vi "Receiver UI.vi"(8 "Error In":errorcluster) -> (0 "Error Out":errorcluster, 11 "Notification":bool)   [LabVIEW 2020, in "Receiver.lvclass"]
doc: "The VI receives data from sender and displays the received message of different data types."
uses:
  Receiver.lvclass
  Controls/Queue Operation.ctl
  Controls/User Event Operations.ctl
  Controls/Receiver Data.ctl
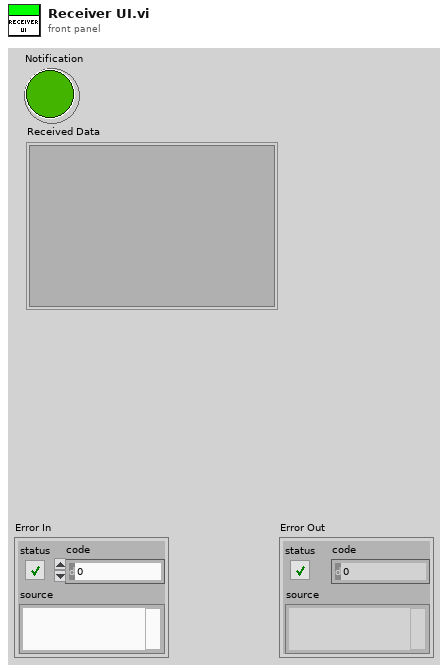
[diagram p1: front panel]
types:
  T1 = typedef "Receiver Data.ctl" = cluster{"Notification":bool}
  T2 = typedef "User Event Operations.ctl" = enum16{"Obtain", "Generate", "Destroy"}
  T3 = typedef "Queue Operation.ctl" = enum16{"Create & Enqueue N", "Enqueue N", "Dequeue", "Enstack N", "Flush", "Release"}
  T4 = typedef "Queue Element.ctl" = cluster{"State":string, "Data":variant}
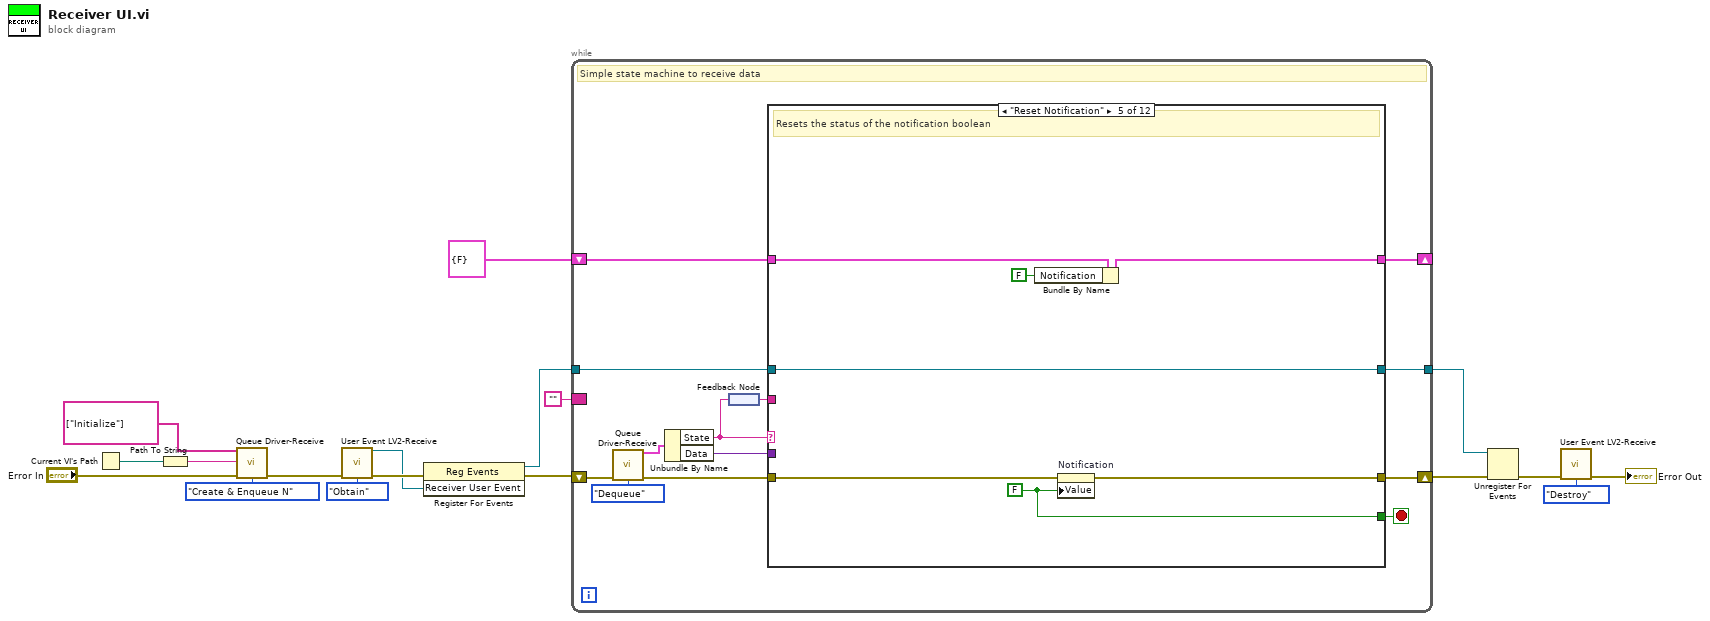
[diagram p0: block diagram]
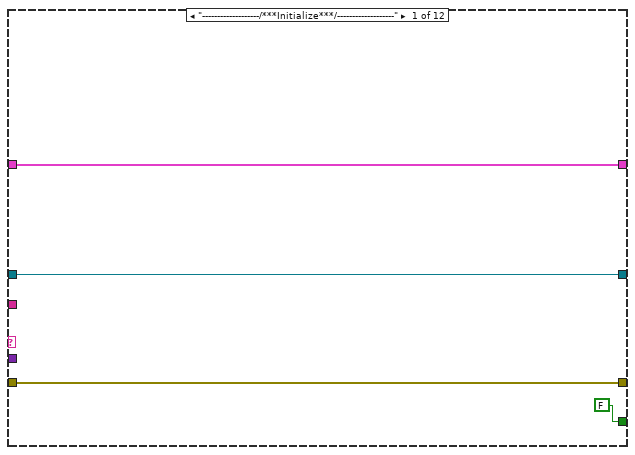
[diagram p2: hidden frame]
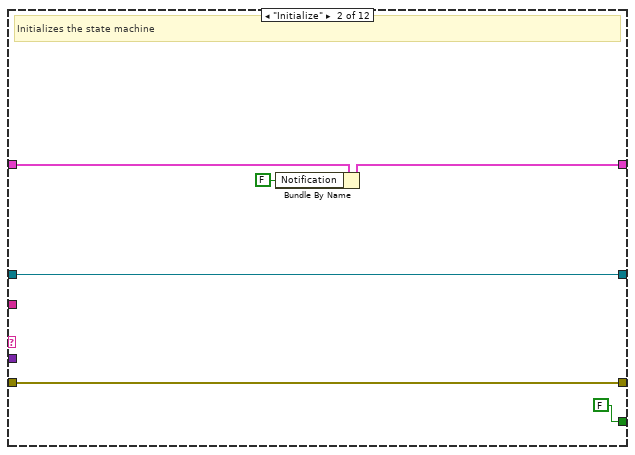
[diagram p3: hidden frame]
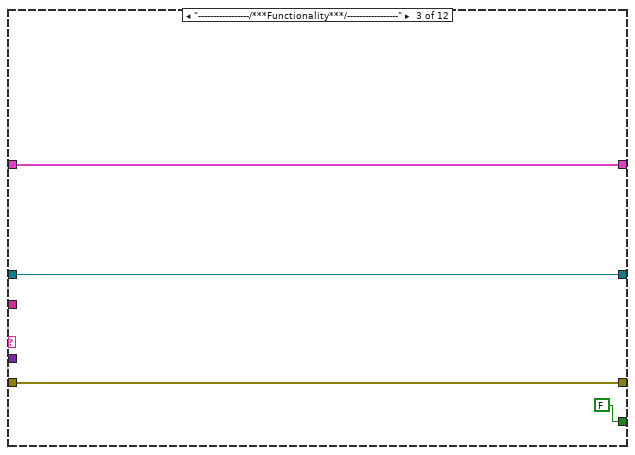
[diagram p4: hidden frame]
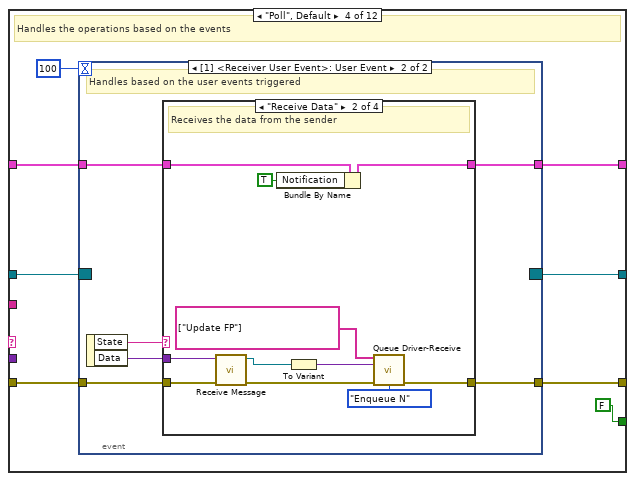
[diagram p5: hidden frame]
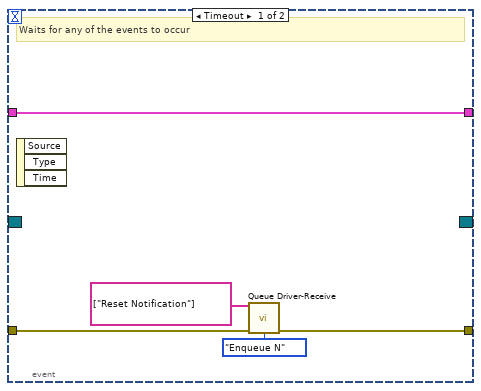
[diagram p6: hidden frame]
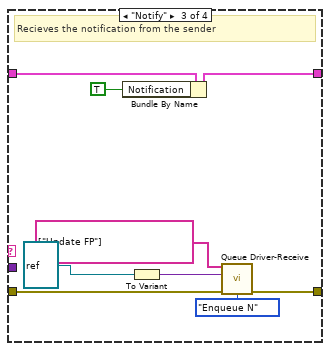
[diagram p8: hidden frame]
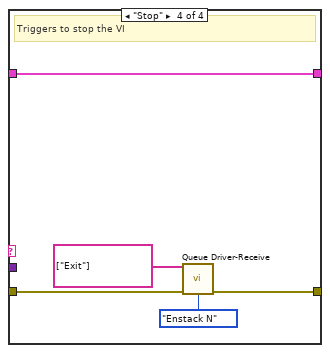
[diagram p9: hidden frame]
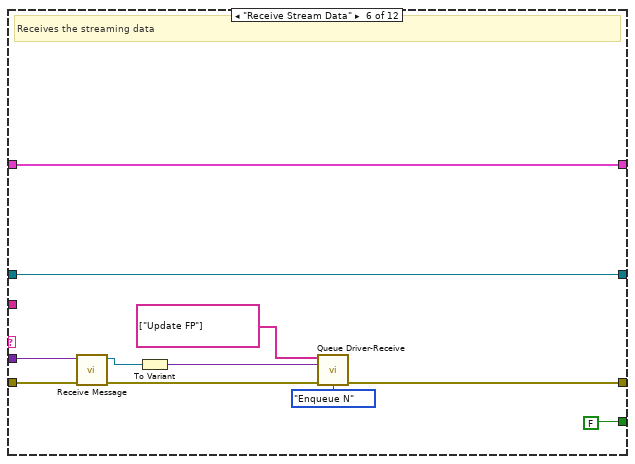
[diagram p10: hidden frame]
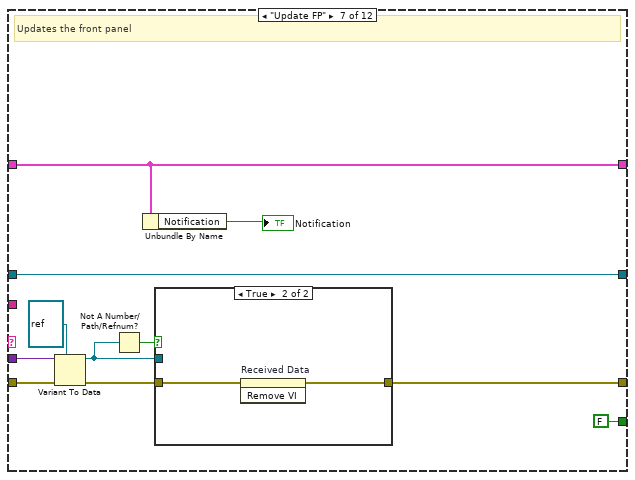
[diagram p11: hidden frame]
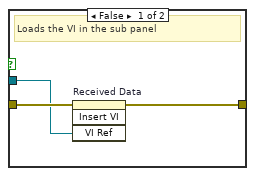
[diagram p12: hidden frame]
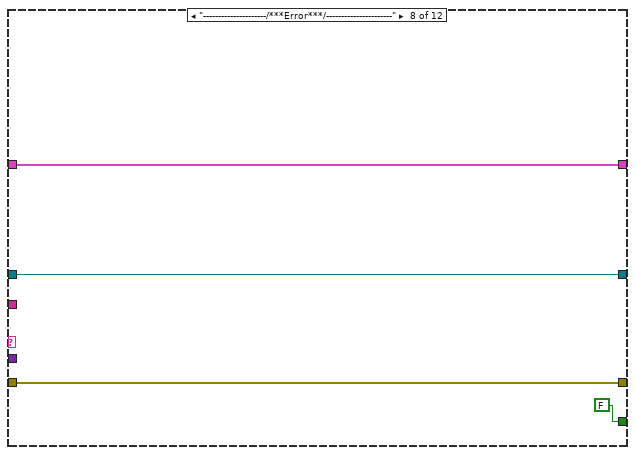
[diagram p13: hidden frame]
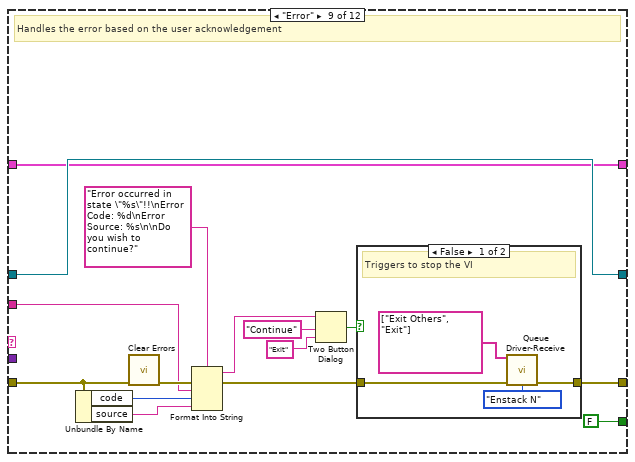
[diagram p14: hidden frame]
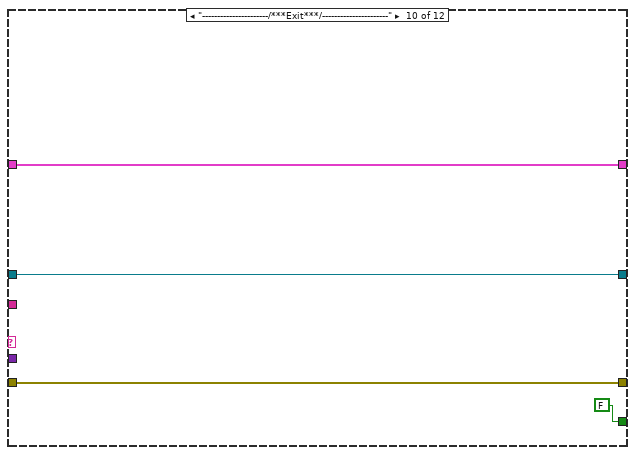
[diagram p16: hidden frame]
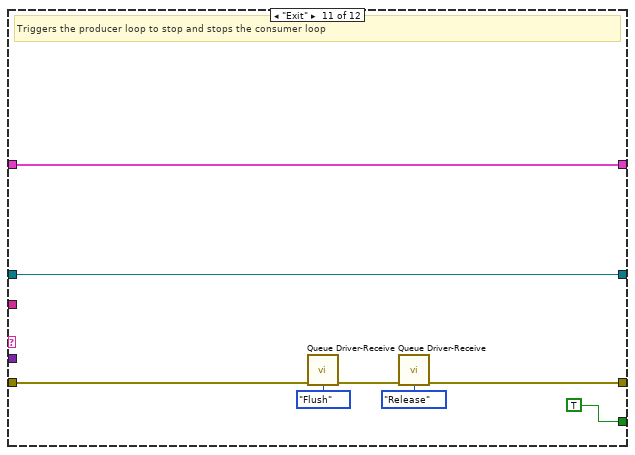
[diagram p17: hidden frame]
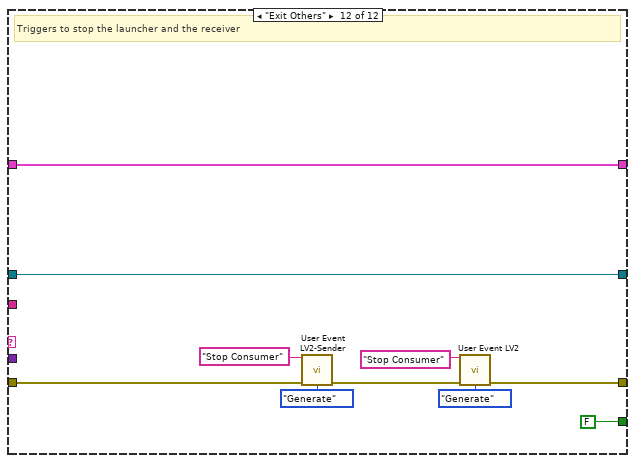
[diagram p18: hidden frame]
diagram:
  n1 = Current VI's Path() -> (path=w3:path)
  n2 = Path To String(path=w3) -> (string=w2:string)
  n3 = call "Queue Driver-Receive.vi"("States[]"=string[] ["Initialize"], "Queue Name"=w2, "Error In"="Error In", "Queue Operation"=Queue_Operation."Create & Enqueue N") -> ("Error Out"=w15:errorcluster)  [unwired: 10 in, 1 out]
  n4 = call "User Event LV2-Receive.vi"("Error In"=w15, "Operation"=User_Event_Operations."Obtain") -> ("Receiver User Event"=w9:refnum<user-event>, "Error Out"=w12:errorcluster)  [unwired: 12 in]
  n5 = register-events(error in=w12, w9) -> (reference out=w8:refnum<event-registration>, error out=w10:errorcluster)  [unwired: 1 in]
  n6 = while {
    shift-right: [w30] -> w16
    shift-left: w10 -> [w31]
    border: "" -> [_]
    tunnel: w8 -> [w23]
    tunnel: [w22] -> w6
    shift-right: [w19] -> _
    shift-left: T1 {"Notification"=FALSE} ("Receiver Data") -> [w20]
    stop <- w27 stop-if-true
    # "Simple state machine to receive data"
    n7 = call "Queue Driver-Receive.vi"("Error In"=w31, "Queue Operation"=Queue_Operation."Dequeue") -> ("Dequeue Element"=w21:T4, "Error Out"=w29:errorcluster)  [unwired: 12 in]
    n8 = Unbundle By Name(w21) -> ("State"=w26:string, "Data"=w24:variant)
    n9 = feedback-in #1(w26) -> ()
    n10 = feedback #1() -> (w25:string)
    n11 = case shown="\"Reset Notification\"" w26 {
      tunnel: w29 -> [w35 w40 w45 w53 w98 w104 w118 w129 w136 w153 w161 w171]
      tunnel: [w35 w40 w45 w51 w96 w107 w117 w129 w133 w153 w157 w166] -> w30
      tunnel: [FALSE FALSE FALSE FALSE w95 FALSE FALSE FALSE FALSE FALSE TRUE FALSE ("Notification")] -> w27
      tunnel: w25 -> [_ _ _ _ _ _ _ _ w134 _ _ _]
      tunnel: w24 -> [_ _ _ _ _ w102 w115 _ _ _ _ _]
      tunnel: w23 -> [w33 w39 w43 w49 w97 w108 w119 w127 w131 w151 w155 w170]
      tunnel: [w33 w39 w43 w48 w97 w108 w119 w127 w131 w151 w155 w170] -> w22
      tunnel: w20 -> [w32 w38 w42 w47 w94 w99 w111 w126 w130 w150 w154 w162]
      tunnel: [w32 w37 w42 w46 w93 w99 w111 w126 w130 w150 w154 w162] -> w19
      frame "-------------------/***Initialize***/-------------------" {
      }
      frame "Initialize" {
        # "Initializes the state machine"
        n12 = Bundle By Name(cluster=w38, "Notification"=FALSE) -> (w37:T1)
      }
      frame "-----------------/***Functionality***/-----------------" {
      }
      frame "Poll", Default {
        # "Handles the operations based on the events"
        n13 = event shown="[1] <Receiver User Event>: User Event" {
          selector: w49 -> [_ _]
          dyn-events: [_ _] -> w48
          timeout: 100 -> [_ _]
          tunnel: w53 -> [w58 w64]
          tunnel: [w57 w63] -> w51
          tunnel: w47 -> [w54 w60]
          tunnel: [w54 w59] -> w46
          event Timeout {
            # "Waits for any of the events to occur"
            n14 = event-data() -> ()  [unwired: 1 in, 3 out]
            n15 = call "Queue Driver-Receive.vi"("States[]"=string[] ["Reset Notification"], "Error In"=w58, "Queue Operation"=Queue_Operation."Enqueue N") -> ("Error Out"=w57:errorcluster)  [unwired: 11 in, 1 out]
          }
          event User Event {
            # "Handles based on the user events triggered"
            n16 = event-data() -> ("State"=w62:string, "Data"=w61:variant)  [unwired: 1 in]
            n17 = case shown="\"Receive Data\"" w62 {
              tunnel: w64 -> [w66 w77 w86 w91]
              tunnel: [w66 w74 w85 w90] -> w63
              tunnel: w61 -> [_ w75 _ _]
              tunnel: w60 -> [w65 w69 w80 w87]
              tunnel: [w65 w68 w79 w87] -> w59
              frame Default {
                # "Do nothing"
              }
              frame "Receive Data" {
                # "Receives the data from the sender"
                n18 = call "Receive Message.vi"("Error In"=w77, "Data"=w75) -> ("Error Out"=w76:errorcluster, "Display Ref"=w71:refnum<vi>)  [unwired: 8 in]
                n19 = Bundle By Name(cluster=w69, "Notification"=TRUE) -> (w68:T1)
                n20 = To Variant(anything=w71) -> (Variant=w73:variant)
                n21 = call "Queue Driver-Receive.vi"("States[]"=string[] ["Update FP"], "Data"=w73, "Error In"=w76, "Queue Operation"=Queue_Operation."Enqueue N") -> ("Error Out"=w74:errorcluster)  [unwired: 10 in, 1 out]
              }
              frame "Notify" {
                # "Recieves the notification from the sender"
                n22 = Bundle By Name(cluster=w80, "Notification"=TRUE) -> (w79:T1)
                n23 = To Variant(anything=refnum<vi> refnum ("VI Ref")) -> (Variant=w81:variant)
                n24 = call "Queue Driver-Receive.vi"("States[]"=string[] ["Update FP"], "Data"=w81, "Error In"=w86, "Queue Operation"=Queue_Operation."Enqueue N") -> ("Error Out"=w85:errorcluster)  [unwired: 10 in, 1 out]
              }
              frame "Stop" {
                # "Triggers to stop the VI"
                n25 = call "Queue Driver-Receive.vi"("States[]"=string[] ["Exit"], "Error In"=w91, "Queue Operation"=Queue_Operation."Enstack N") -> ("Error Out"=w90:errorcluster)  [unwired: 11 in, 1 out]
              }
            }
          }
        }
      }
      frame "Reset Notification" {
        w95 = FALSE ("Notification")
        # "Resets the status of the notification boolean"
        n26 = Bundle By Name(cluster=w94, "Notification"=FALSE) -> (w93:T1)
        n27 = property on="Notification" class="Bool (strict)"(error in=w98, "Value"=w95) -> (error out=w96:errorcluster)  [unwired: 1 in, 1 out]
      }
      frame "Receive Stream Data" {
        # "Receives the streaming data"
        n28 = call "Receive Message.vi"("Error In"=w104, "Data"=w102) -> ("Error Out"=w103:errorcluster, "Display Ref"=w100:refnum<vi>)  [unwired: 8 in]
        n29 = To Variant(anything=w100) -> (Variant=w101:variant)
        n30 = call "Queue Driver-Receive.vi"("States[]"=string[] ["Update FP"], "Data"=w101, "Error In"=w103, "Queue Operation"=Queue_Operation."Enqueue N") -> ("Error Out"=w107:errorcluster)  [unwired: 10 in, 1 out]
      }
      frame "Update FP" {
        # "Updates the front panel"
        n31 = Variant To Data(error in=w118, type=refnum<vi> refnum ("VI Ref"), Variant=w115) -> (data=w113:refnum<vi>, error out=w116:errorcluster)
        n32 = Not A Number/Path/Refnum?(number/path/refnum=w113) -> (NaN/Path/Refnum?=w112:bool)
        n33 = Unbundle By Name(w111) -> ("Notification"=→"Notification":bool)
        n34 = case shown="True" w112 {
          tunnel: [w123 w124] -> w117
          tunnel: w116 -> [w122 w125]
          tunnel: w113 -> [w121 _]
          frame False {
            # "Loads the VI in the sub panel"
            n35 = invoke on="Received Data" class="SubPnl" method="Insert VI"(error in=w122, "VI Ref"=w121) -> (error out=w123:errorcluster)  [unwired: 2 in, 3 out]
          }
          frame True {
            n36 = invoke on="Received Data" class="SubPnl" method="Remove VI"(error in=w125) -> (error out=w124:errorcluster)  [unwired: 2 in, 2 out]
          }
        }
      }
      frame "---------------------/***Error***/----------------------" {
      }
      frame "Error" {
        # "Handles the error based on the user acknowledgement"
        n37 = Unbundle By Name(w136) -> ("code"=w138:i32, "source"=w137:string)
        n38 = call <vilib>:"Clear Errors.vi"("error in (no error)"=w136) -> ("error out"=w143:errorcluster)  [unwired: 5 in, 1 out]
        n39 = Format Into String(format string="Error occurred in state \"%s\"!!\nError Code: %d\nError Source: %s\n\nDo you wish to continue?", error in=w143, w134, w138, w137) -> (resulting string=w141:string, error out=w135:errorcluster)  [unwired: 1 in]
        n40 = Two Button Dialog(message=w141, 1:"Exit" ("F button name (\"Cancel\")"), 2:"Continue" ("T button name (\"OK\")")) -> (T button?=w132:bool)
        n41 = case shown="False" w132 {
          tunnel: w135 -> [w148 w149]
          tunnel: [w147 w149] -> w133
          frame False {
            # "Triggers to stop the VI"
            n42 = call "Queue Driver-Receive.vi"("States[]"=string[] ["Exit Others", "Exit"], "Error In"=w148, "Queue Operation"=Queue_Operation."Enstack N") -> ("Error Out"=w147:errorcluster)  [unwired: 11 in, 1 out]
          }
          frame True {
          }
        }
      }
      frame "----------------------/***Exit***/----------------------" {
      }
      frame "Exit" {
        # "Triggers the producer loop to stop and stops the consumer loop"
        n43 = call "Queue Driver-Receive.vi"("Error In"=w161, "Queue Operation"=Queue_Operation."Flush") -> ("Error Out"=w159:errorcluster)  [unwired: 12 in, 1 out]
        n44 = call "Queue Driver-Receive.vi"("Error In"=w159, "Queue Operation"=Queue_Operation."Release") -> ("Error Out"=w157:errorcluster)  [unwired: 12 in, 1 out]
      }
      frame "Exit Others" {
        # "Triggers to stop the launcher and the receiver"
        n45 = call "User Event LV2-Sender.vi"("Event Name"="Stop Consumer", "Error In"=w171, "Operation"=User_Event_Operations."Generate") -> ("Error Out"=w168:errorcluster)  [unwired: 11 in, 1 out]
        n46 = call "User Event LV2.vi"("Event Name"="Stop Consumer", "Error In"=w168, "Operation"=User_Event_Operations."Generate") -> ("Error Out"=w166:errorcluster)  [unwired: 11 in, 1 out]
      }
    }
  }
  n47 = Unregister For Events(event registration refnum=w6, error in=w16) -> (error out=w7:errorcluster)
  n48 = call "User Event LV2-Receive.vi"("Error In"=w7, "Operation"=User_Event_Operations."Destroy") -> ("Error Out"=→"Error Out":errorcluster)  [unwired: 12 in, 1 out]
